vi "Info from Folder.vi"(8 "error in (no error)":errorcluster, 9 "Name":string, 10 "Folder":path, 11 "NamedPackage in":refnum<class "NamedPackage.lvclass">) -> (0 "error out":errorcluster, 2 "Package Info":T1)   [LabVIEW 2020, in "GPack.lvlib" / "NamedPackage.lvclass"]
uses:
  NamedPackage.lvclass
  Package Info.ctl
  GPack.lvlib
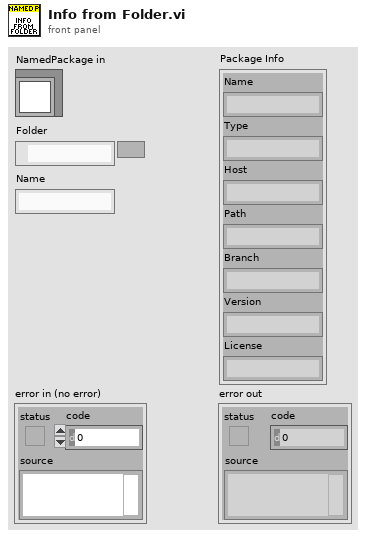
[diagram p1: front panel]
types:
  T1 = typedef "GPack.lvlib/Package Info.ctl" = cluster{"Name":string, "Type":string, "Host":string, "Path":string, "Branch":string, "Version":string, "License":string}
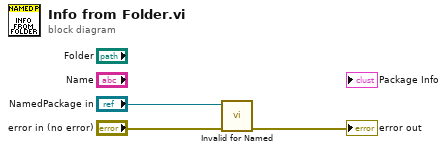
[diagram p0: block diagram]
diagram:
  n1 = call "Invalid for Named.vi"("error in (no error)"="error in (no error)", "NamedPackage in"="NamedPackage in") -> ("error out"=→"error out":errorcluster)  [unwired: 8 in, 1 out]
